vi "zmq stopwatch stop.vi"(8 "error in (no error)":errorcluster, 11 "watch_":u32) -> (0 "error out":errorcluster, 2 "function return":u32, 3 "watch_ out":u32)   [LabVIEW 2025, in "LibZMQ.lvlib"]
doc: "ZMQ_EXPORT unsigned long zmq_stopwatch_stop (void *watch_);"
uses:
  LibZMQ.lvlib
  LV/LibZMQ/libzmq/lv_x86/bin/Release/libzmq-v143-mt-4_3_6.dll
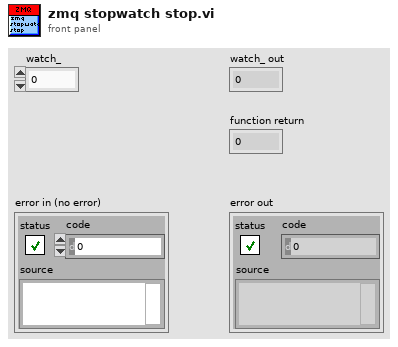
[diagram p1: front panel]
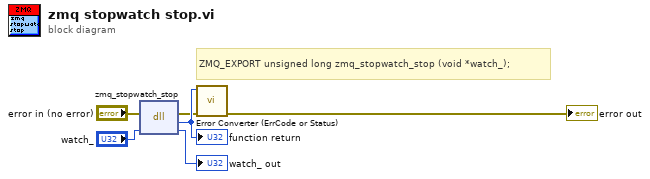
[diagram p0: block diagram]
diagram:
  # "ZMQ_EXPORT unsigned long zmq_stopwatch_stop (void *watch_);"
  n1 = dll-call lib="C:/LV/LibZMQ/libzmq/lv_x86/bin/Release/libzmq-v143-mt-4_3_6.*" fn="zmq_stopwatch_stop"(error in="error in (no error)", "watch_"="watch_") -> (error out=w2:errorcluster, w6:u32, "watch_"=→"watch_ out":u32)  [unwired: 2 in, 1 out]
  "function return" <- w6
  n2 = call "Error Converter (ErrCode or Status).vi"("error in (no error)"=w2, "error code"=w6) -> ("error out"=→"error out":errorcluster)  [unwired: 9 in]
